vi "umToslmRadius.vi"(1 "z (um)":dbl) -> (0 "hologram radius (pixels)":i32)   [LabVIEW 2020]
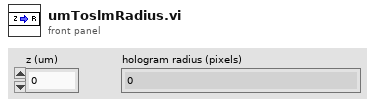
[diagram p1: front panel]
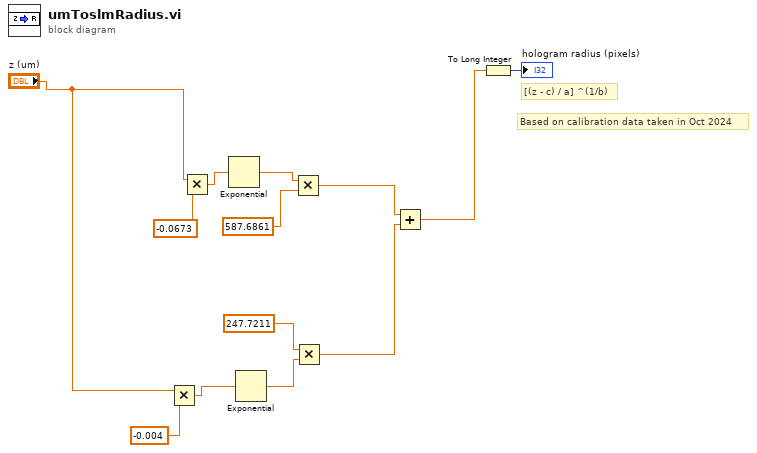
[diagram p0: block diagram]
diagram:
  # "Based on calibration data taken in Oct 2024"
  # "[(z - c) / a] ^(1/b)"
  n1 = Multiply(x="z (um)", y=-0.004) -> (x*y=w5:dbl)
  n2 = Multiply(x="z (um)", y=-0.0673) -> (x*y=w12:dbl)
  n3 = Exponential(1:w12) -> (0:w9:dbl)
  n4 = Exponential(1:w5) -> (0:w4:dbl)
  n5 = Multiply(x=w9, y=587.6861) -> (x*y=w8:dbl)
  n6 = Multiply(x=247.7211, y=w4) -> (x*y=w2:dbl)
  n7 = Add(x=w8, y=w2) -> (x+y=w1:dbl)
  n8 = To Long Integer(number=w1) -> (32bit integer=→"hologram radius (pixels)":i32)
